vi "GetTestDataHeader.vi"(7 "Boolean":bool, 11 "TESTPLAN ARRAY":string[][](array[string])=[["CUSTOMER P/N:", "SCR-Relay IDM20A", "", "", "", "", "", "", "", "", "", "", "", ""], ["SVI P/N:", "SAB213-143LF", "", "", "", "", "", "", "", "", "", "", "", ""], ["CREATED DATE:", "12-ÁÕ.¤.-14", "", "", "", "", "", "", "", "", "", "", "", ""], ["SW REV.:", "1.000", "", "", "", "", "", "", "", "", "", "", "", ""], ["TEST SEQ REV.:", "1.000", "", "", "", "", "", "", "", "", "", "", "", ""], ["Index", " Step#", "Descriptions", "FailedCode", "Equipment", "Command", "Action ", "Low Limit", "High Limit", "Unit", "Test Loop", "Compensate", "Remarks", "RLY Status"], ["1", "0", "Initial", "", "", "", "STEP", "", "", "", "", "", "", ""], ["2", "", "Clear all relays", "", "RELAY", "@b000t", "TEST", "", "", "", "", "", "", ""], ["3", "1", "Test of Transformer", "", "", "", "STEP", "", "", "", "", "", "", ""], ["4", "", "\"ON RLY1,2 to connect 230VAC to X11-1(L) and X11-3(N)\"", "", "RELAY", "@b001t", "TEST", "", "", "", "", "", "", "\"1,2\""], ["5", "", "Check for 24-30 VAC between X14.1-2.", "", "", "", "STEP", "", "", "", "", "", "", ""], ["6", "", "CONF 34450A to meas. VAC", "", "34450A", "CONF:VOLT:AC 750", "TEST", "", "", "", "", "", "", ""], ["7", "", "\"ON RLY14, 15 to connect 34450A to meas 24VAC\"", "", "RELAY", "@b011t", "TEST", "", "", "", "", "", "", "\"1,2,14,15\""], ["8", "", "Meas 24VAC at X14-1 and X14-2", "1.1", "34450A", "READ?", "TEST", "24", "30", "VAC", "", "", "", ""], ["9", "", "Delay 250mS", "", "DELAY", "250", "TEST", "", "", "", "", "", "", ""], ["10", "2", "Check of PTC-resistors", "", "", "", "STEP", "", "", "", "", "", "", ""], ["11", "", "\"35R at X14-1 & 2, 24VAC at X14-1&2 < 17VAC after 10 sec\"", "2.1", "34450A", "PTC-V35R", "TEST", "10", "15", "Sec", "", "", "35R is connected here in a routine", "\"1,2,14,15,12,13\""], ["12", "", "\"OFF RLY12, 13 to disconnect 35R from X14-1 and X14-2\"", "", "RELAY", "@b010f", "TEST", "", "", "", "", "", "", "\"1,2,14,15\""], ["13", "", "\"OFF RLY14, 15 to disconnect 34450A from X14-1 and X14-2\"", "", "RELAY", "@b011f", "TEST", "", "", "", "", "", "", "\"1,2\""], ["14", "", "CONF 34450A to meas. IAC", "", "34450A", "CONF:CURR:AC 1", "TEST", "", "", "", "", "", "", ""], ["15", "", "\"15R & AC-AMP at X14-1 & 2, I thru 15R <100mA in 15 Sec\"", "2.2", "34450A", "PTC-I15R", "TEST", "15", "20", "Sec", "", "", "15R is connected here in a routine", "\"1,2,16,17,18\""], ["16", "", "\"OFF RLY16,17,18 to disconnect 15R and AC-AMP from X14-1 & 2\"", "", "RELAY", "@b012f", "TEST", "", "", "", "", "", "", "\"1,2\""], ["17", "3", "Test of +34 Volt", "", "", "", "STEP", "", "", "", "", "", "", ""], ["18", "", "CONF 34450A to meas. VDC", "", "34450A", "CONF:VOLT:DC 100", "TEST", "", "", "", "", "", "", ""], ["19", "", "\"ON RLY19,20 to connect 34450A to +34V and GND (X13-8)\"", "", "RELAY", "@b013t", "TEST", "", "", "", "", "", "", "\"1,2,19,20\""], ["20", "", "Meas +34 Volt", "3.1", "34450A", "READ?", "TEST", "30", "38", "VDC", "", "", "", ""], ["21", "", "\"OFF RLY19,20 to disconnect 34450A from +34V and GND (X13-8)\"", "", "RELAY", "@b013t", "TEST", "", "", "", "", "", "", "\"1,2\""], ["22", "", "Test of relays: ", "", "", "", "STEP", "", "", "", "", "", "", ""], ["23", "4", "Test of K1", "", "", "", "STEP", "", "", "", "", "", "", ""], ["24", "", "LED9 is OFF?", "4.1", "MESSAGE", "", "TEST", "1", "1", "", "", "", "", ""], ["25", "", "ON RLY21 to connect 16mA curr to X13-3", "", "RELAY", "@b014t", "TEST", "", "", "", "", "", "", "\"1,2,21\""], ["26", "", "\"ON RLY24,25 to connect 34450A to GND of 16mA CON CKT and X13-1\"", "", "RELAY", "@b017t", "TEST", "", "", "", "", "", "", "\"1,2,21,24,25\""], ["27", "", "Meas VX13-1", "4.2", "34450A", "READ?", "TEST", "-0.5", "0.5", "VDC", "", "", "", ""], ["28", "", "\"OFF RLY24,25 to disconnect 34450A from GND of 16mA CON CKT and X13-1\"", "", "RELAY", "@b017f", "TEST", "", "", "", "", "", "", "\"1,2,21\""], ["29", "", "\"ON RLY24,26 to connect 34450A to GND of 16mA CON CKT and X13-2\"", "", "RELAY", "@b018t", "TEST", "", "", "", "", "", "", "\"1,2,21,24,26\""], ["30", "", "Meas VX13-2", "4.3", "34450A", "READ?", "TEST", "7", "8", "VDC", "", "", "", ""], ["31", "", "\"OFF RLY24,26 to disconnect 34450A from GND of 16mA CON CKT and X13-2\"", "", "RELAY", "@b018f", "TEST", "", "", "", "", "", "", "\"1,2,21\""], ["32", "", "ON RLY5 to activate K1", "", "RELAY", "@b003t", "TEST", "", "", "", "", "", "", "\"1,2,5,21\""], ["33", "", "LED9 is ON?", "4.4", "MESSAGE", "", "TEST", "1", "1", "", "", "", "", ""], ["34", "", "\"ON RLY24,25 to connect 34450A to GND of 16mA CON CKT and X13-1\"", "", "RELAY", "@b017t", "TEST", "", "", "", "", "", "", "\"1,2,5,21,24,25\""], ["35", "", "Meas VX13-1", "4.5", "34450A", "READ?", "TEST", "7", "8", "VDC", "", "", "", ""], ["36", "", "\"OFF RLY24,25 to disconnect 34450A from GND of 16mA CON CKT and X13-1\"", "", "RELAY", "@b017f", "TEST", "", "", "", "", "", "", "\"1,2,5,21\""], ["37", "", "\"ON RLY24,26 to connect 34450A to GND of 16mA CON CKT and X13-2\"", "", "RELAY", "@b018t", "TEST", "", "", "", "", "", "", "\"1,2,5,21,24,26\""], ["38", "", "Meas VX13-2", "4.6", "34450A", "READ?", "TEST", "-0.5", "0.5", "VDC", "", "", "", ""], ["39", "", "\"OFF RLY24,26 to disconnect 34450A from GND of 16mA CON CKT and X13-2\"", "", "RELAY", "@b018f", "TEST", "", "", "", "", "", "", "\"1,2,5,21\""], ["40", "", "OFF RLY21 to disconnect 16mA curr from X13-3", "", "RELAY", "@b014f", "TEST", "", "", "", "", "", "", "\"1,2,5\""], ["41", "", "OFF RLY5 to de-activate K1", "", "RELAY", "@b003f", "TEST", "", "", "", "", "", "", "\"1,2\""], ["42", "5", "Test of K2", "", "", "", "STEP", "", "", "", "", "", "", ""], ["43", "", "LED10 is OFF?", "5.1", "MESSAGE", "", "TEST", "1", "1", "", "", "", "", ""], ["44", "", "ON RLY22 to connect 16mA curr to X13-6", "", "RELAY", "@b015t", "TEST", "", "", "", "", "", "", "\"1,2,22\""], ["45", "", "\"ON RLY24,27 to connect 34450A to GND of 16mA CON CKT and X13-4\"", "", "RELAY", "@b019t", "TEST", "", "", "", "", "", "", "\"1,2,22,24,27\""], ["46", "", "Meas VX13-4", "5.2", "34450A", "READ?", "TEST", "-0.5", "0.5", "VDC", "", "", "", ""], ["47", "", "\"OFF RLY24,27 to disconnect 34450A from GND of 16mA CON CKT and X13-4\"", "", "RELAY", "@b019f", "TEST", "", "", "", "", "", "", "\"1,2,22\""], ["48", "", "\"ON RLY24,28 to connect 34450A to GND of 16mA CON CKT and X13-5\"", "", "RELAY", "@b020t", "TEST", "", "", "", "", "", "", "\"1,2,22,24,28\""], ["49", "", "Meas VX13-5", "5.3", "34450A", "READ?", "TEST", "7", "8", "VDC", "", "", "", ""], ["50", "", "\"OFF RLY24,28 to disconnect 34450A from GND of 16mA CON CKT and X13-5\"", "", "RELAY", "@b020f", "TEST", "", "", "", "", "", "", "\"1,2,22\""], ["51", "", "ON RLY6 to activate K2", "", "RELAY", "@b004t", "TEST", "", "", "", "", "", "", "\"1,2,4,22\""], ["52", "", "LED10 is ON?", "5.4", "MESSAGE", "", "TEST", "1", "1", "", "", "", "", ""], ["53", "", "\"ON RLY24,27 to connect 34450A to GND of 16mA CON CKT and X13-4\"", "", "RELAY", "@b019t", "TEST", "", "", "", "", "", "", "\"1,2,4,22,24,27\""], ["54", "", "Meas VX13-4", "5.2", "34450A", "READ?", "TEST", "7", "8", "VDC", "", "", "", ""], ["55", "", "\"OFF RLY24,27 to disconnect 34450A from GND of 16mA CON CKT and X13-4\"", "", "RELAY", "@b019f", "TEST", "", "", "", "", "", "", "\"1,2,4,22\""], ["56", "", "\"ON RLY24,28 to connect 34450A to GND of 16mA CON CKT and X13-5\"", "", "RELAY", "@b020t", "TEST", "", "", "", "", "", "", "\"1,2,4,22,24,28\""], ["57", "", "Meas VX13-5", "5.3", "34450A", "READ?", "TEST", "-0.5", "0.5", "VDC", "", "", "", ""], ["58", "", "\"OFF RLY24,28 to disconnect 34450A from GND of 16mA CON CKT and X13-5\"", "", "RELAY", "@b020f", "TEST", "", "", "", "", "", "", "\"1,2,4,22\""], ["59", "", "OFF RLY22 to disconnect 16mA curr from X13-6", "", "RELAY", "@b015f", "TEST", "", "", "", "", "", "", "\"1,2,4\""], ["60", "", "OFF RLY6 to de-activate K2", "", "RELAY", "@b004f", "TEST", "", "", "", "", "", "", "\"1,2\""], ["61", "6", "Test of K3", "", "", "", "STEP", "", "", "", "", "", "", ""], ["62", "", "LED11 is OFF?", "6.1", "MESSAGE", "", "TEST", "1", "1", "", "", "", "", ""], ["63", "", "ON RLY23 to connect 16mA curr to X13-8", "", "RELAY", "@b016t", "TEST", "", "", "", "", "", "", "\"1,2,23\""], ["64", "", "\"ON RLY24,29 to connect 34450A to GND of 16mA CON CKT and X13-7\"", "", "RELAY", "@b021t", "TEST", "", "", "", "", "", "", "\"1,2,23,24,29\""], ["65", "", "Meas VX13-7", "6.2", "34450A", "READ?", "TEST", "-0.5", "0.5", "VDC", "", "", "", ""], ["66", "", "\"OFF RLY24,29 to disconnect 34450A from GND of 16mA CON CKT and X13-7\"", "", "RELAY", "@b021f", "TEST", "", "", "", "", "", "", "\"1,2,23\""], ["67", "", "\"ON RLY24,35 to connect 34450A to GND of 16mA CON CKT and X13-9\"", "", "RELAY", "@b029t", "TEST", "", "", "", "", "", "", "\"1,2,23,24,35\""], ["68", "", "Meas VX13-9", "6.3", "34450A", "READ?", "TEST", "7", "8", "VDC", "", "", "", ""], ["69", "", "\"OFF RLY24,35 to disconnect 34450A from GND of 16mA CON CKT and X13-9\"", "", "RELAY", "@b029f", "TEST", "", "", "", "", "", "", "\"1,2,23\""], ["70", "", "ON RLY7 to activate K3", "", "RELAY", "@b005t", "TEST", "", "", "", "", "", "", "\"1,2,3,23\""], ["71", "", "LED11 is ON?", "6.4", "MESSAGE", "", "TEST", "1", "1", "", "", "", "", ""], ["72", "", "\"ON RLY24,29 to connect 34450A to GND of 16mA CON CKT and X13-7\"", "", "RELAY", "@b021t", "TEST", "", "", "", "", "", "", "\"1,2,23,24,29\""], ["73", "", "Meas VX13-7", "6.2", "34450A", "READ?", "TEST", "7", "8", "VDC", "", "", "", ""], ["74", "", "\"OFF RLY24,29 to disconnect 34450A from GND of 16mA CON CKT and X13-7\"", "", "RELAY", "@b021f", "TEST", "", "", "", "", "", "", "\"1,2,23\""], ["75", "", "\"ON RLY24,35 to connect 34450A to GND of 16mA CON CKT and X13-9\"", "", "RELAY", "@b029t", "TEST", "", "", "", "", "", "", "\"1,2,23,24,35\""], ["76", "", "Meas VX13-9", "6.3", "34450A", "READ?", "TEST", "-0.5", "0.5", "VDC", "", "", "", ""], ["77", "", "\"OFF RLY24,35 to disconnect 34450A from GND of 16mA CON CKT and X13-9\"", "", "RELAY", "@b029f", "TEST", "", "", "", "", "", "", "\"1,2,23\""], ["78", "", "OFF RLY23 to disconnect 16mA curr from X13-3", "", "RELAY", "@b016f", "TEST", "", "", "", "", "", "", "\"1,2,3\""], ["79", "", "OFF RLY5 to de-activate K1", "", "RELAY", "@b005f", "TEST", "", "", "", "", "", "", "\"1,2\""], ["80", "", "Test of SC-relay", "", "", "", "STEP", "", "", "", "", "", "", ""], ["81", "7", "Test of TI4", "", "", "", "STEP", "", "", "", "", "", "", ""], ["82", "", "CONF 34450A to meas. VAC", "", "34450A", "CONF:VOLT:AC 750", "TEST", "", "", "", "", "", "", ""], ["83", "", "LED8 is OFF?", "7.1", "MESSAGE", "", "TEST", "1", "1", "", "", "", "", ""], ["84", "", "\"ON RLY30,34 to connect 34450A to X12-1 (L) & X11-3 (N)\"", "", "RELAY", "@b022t", "TEST", "", "", "", "", "", "", "\"1,2,30,34\""], ["85", "", "Meas VX12-1 (L) & X11-3 (N)-NoActivated", "7.2", "34450A", "READ?", "TEST", "0", "10", "VAC", "", "", "", ""], ["86", "", "ON RLY8 to activate TI4 (X15-4 to X15-8)", "", "RELAY", "@b006t", "TEST", "", "", "", "", "", "", "\"1,2,30,34,8\""], ["87", "", "Delay 250mS", "", "DELAY", "250", "TEST", "", "", "", "", "", "", ""], ["88", "", "LED8 is ON?", "7.3", "MESSAGE", "", "TEST", "1", "1", "", "", "", "", ""], ["89", "", "Meas VX12-1 (L) & X11-3 (N)-Activated", "7.4", "34450A", "READ?", "TEST", "210", "250", "VAC", "", "", "", ""], ["90", "", "OFF RLY8 to de-activate TI4 (X15-4 to X15-8)", "", "RELAY", "@b006f", "TEST", "", "", "", "", "", "", "\"1,2,30,34\""], ["91", "", "\"OFF RLY30,34 to disconnect 34450A from X12-1 (L) & X11-3 (N)\"", "", "RELAY", "@b022f", "TEST", "", "", "", "", "", "", "\"1,2\""], ["92", "", "Delay 250mS", "", "DELAY", "250", "TEST", "", "", "", "", "", "", ""], ["93", "8", "Test of TI1", "", "", "", "STEP", "", "", "", "", "", "", ""], ["94", "", "LED5 is OFF?", "8.1", "MESSAGE", "", "TEST", "1", "1", "", "", "", "", ""], ["95", "", "\"ON RLY31,34 to connect 34450A to X12-2 (L) & X11-3 (N)\"", "", "RELAY", "@b023t", "TEST", "", "", "", "", "", "", "\"1,2,31,34\""], ["96", "", "Meas VX12-2 (L) & X11-3 (N)-NoActivated", "8.2", "34450A", "READ?", "TEST", "0", "10", "VAC", "", "", "", ""], ["97", "", "ON RLY9 to activate TI1 (X15-5 to X15-8)", "", "RELAY", "@b007t", "TEST", "", "", "", "", "", "", "\"1,2,31,34,9\""], ["98", "", "Delay 250mS", "", "DELAY", "250", "TEST", "", "", "", "", "", "", ""], ["99", "", "LED5 is ON?", "8.3", "MESSAGE", "", "TEST", "1", "1", "", "", "", "", ""], ["100", "", "Meas VX12-2 (L) & X11-3 (N)-Activated", "8.4", "34450A", "READ?", "TEST", "210", "250", "VAC", "", "", "", ""], ["101", "", "OFF RLY9 to de-activate TI1 (X15-5 to X15-8)", "", "RELAY", "@b007f", "TEST", "", "", "", "", "", "", "\"1,2,31,34\""], ["102", "", "\"OFF RLY30,34 to disconnect 34450A from X12-1 (L) & X11-3 (N)\"", "", "RELAY", "@b023f", "TEST", "", "", "", "", "", "", "\"1,2\""], ["103", "", "Delay 250mS", "", "DELAY", "250", "TEST", "", "", "", "", "", "", ""], ["104", "9", "Test of TI2", "", "", "", "STEP", "", "", "", "", "", "", ""], ["105", "", "LED6 is OFF?", "9.1", "MESSAGE", "", "TEST", "1", "1", "", "", "", "", ""], ["106", "", "\"ON RLY32,34 to connect 34450A to X12-3 (L) & X11-3 (N)\"", "", "RELAY", "@b024t", "TEST", "", "", "", "", "", "", "\"1,2,32,34\""], ["107", "", "Meas VX12-3 (L) & X11-3 (N)-NoActivated", "9.2", "34450A", "READ?", "TEST", "0", "10", "VAC", "", "", "", ""], ["108", "", "ON RLY10 to activate TI2 (X15-6 to X15-8)", "", "RELAY", "@b008t", "TEST", "", "", "", "", "", "", "\"1,2,32,34,10\""], ["109", "", "Delay 250mS", "", "DELAY", "250", "TEST", "", "", "", "", "", "", ""], ["110", "", "LED6 is ON?", "9.3", "MESSAGE", "", "TEST", "1", "1", "", "", "", "", ""], ["111", "", "Meas VX12-3 (L) & X11-3 (N)-Activated", "9.4", "34450A", "READ?", "TEST", "210", "250", "VAC", "", "", "", ""], ["112", "", "OFF RLY10 to de-activate TI2 (X15-6 to X15-8)", "", "RELAY", "@b008f", "TEST", "", "", "", "", "", "", "\"1,2,32,34\""], ["113", "", "\"OFF RLY32,34 to disconnect 34450A from X12-3 (L) & X11-3 (N)\"", "", "RELAY", "@b024f", "TEST", "", "", "", "", "", "", "\"1,2\""], ["114", "", "Delay 250mS", "", "DELAY", "250", "TEST", "", "", "", "", "", "", ""], ["115", "10", "Test of TI3", "", "", "", "STEP", "", "", "", "", "", "", ""], ["116", "", "LED7 is OFF?", "10.1", "MESSAGE", "", "TEST", "1", "1", "", "", "", "", ""], ["117", "", "\"ON RLY33,34 to connect 34450A to X12-4 (L) & X11-3 (N)\"", "", "RELAY", "@b025t", "TEST", "", "", "", "", "", "", "\"1,2,33,34\""], ["118", "", "Meas VX12-4 (L) & X11-3 (N)-NoActivated", "10.2", "34450A", "READ?", "TEST", "0", "10", "VAC", "", "", "", ""], ["119", "", "ON RLY11 to activate TI3 (X15-7 to X15-8)", "", "RELAY", "@b009t", "TEST", "", "", "", "", "", "", "\"1,2,33,34,11\""], ["120", "", "Delay 250mS", "", "DELAY", "250", "TEST", "", "", "", "", "", "", ""], ["121", "", "LED7 is ON?", "10.3", "MESSAGE", "", "TEST", "1", "1", "", "", "", "", ""], ["122", "", "Meas VX12-4 (L) & X11-3 (N)-Activated", "10.4", "34450A", "READ?", "TEST", "210", "250", "VAC", "", "", "", ""], ["123", "", "OFF RLY11 to de-activate TI2 (X15-7 to X15-8)", "", "RELAY", "@b009f", "TEST", "", "", "", "", "", "", "\"1,2,33,34\""], ["124", "", "\"OFF RLY33,34 to disconnect 34450A from X12-4 (L) & X11-3 (N)\"", "", "RELAY", "@b025f", "TEST", "", "", "", "", "", "", "\"1,2\""], ["125", "", "Delay 250mS", "", "DELAY", "250", "TEST", "", "", "", "", "", "", ""], ["126", "", "Clear all relays", "", "RELAY", "@b000t", "TEST", "", "", "", "", "", "", ""], ["127", "", "End of testing", "", "", "", "END", "", "", "", "", "", "", ""]]) -> (3 "TestDataHeader":string)   [LabVIEW 2011]
panel:
  out "element 3":i32
  out "size(s)":i32[](array[numeric])
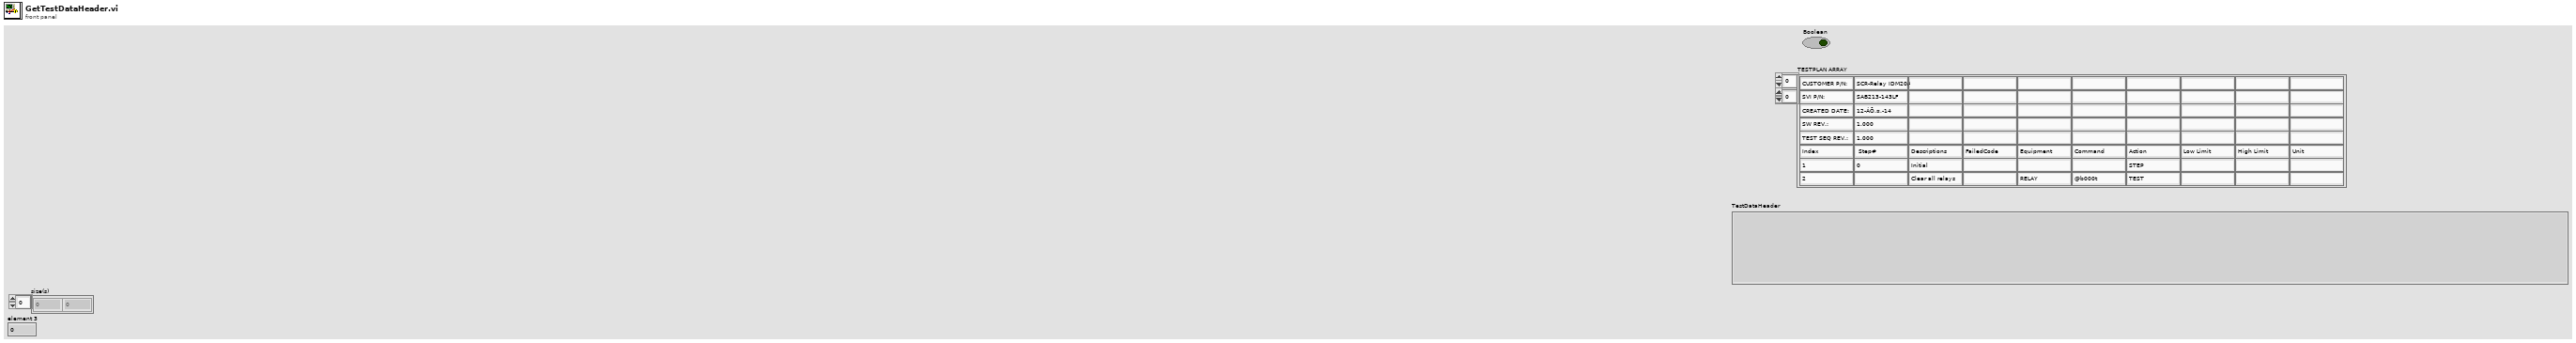
[diagram p1: front panel]
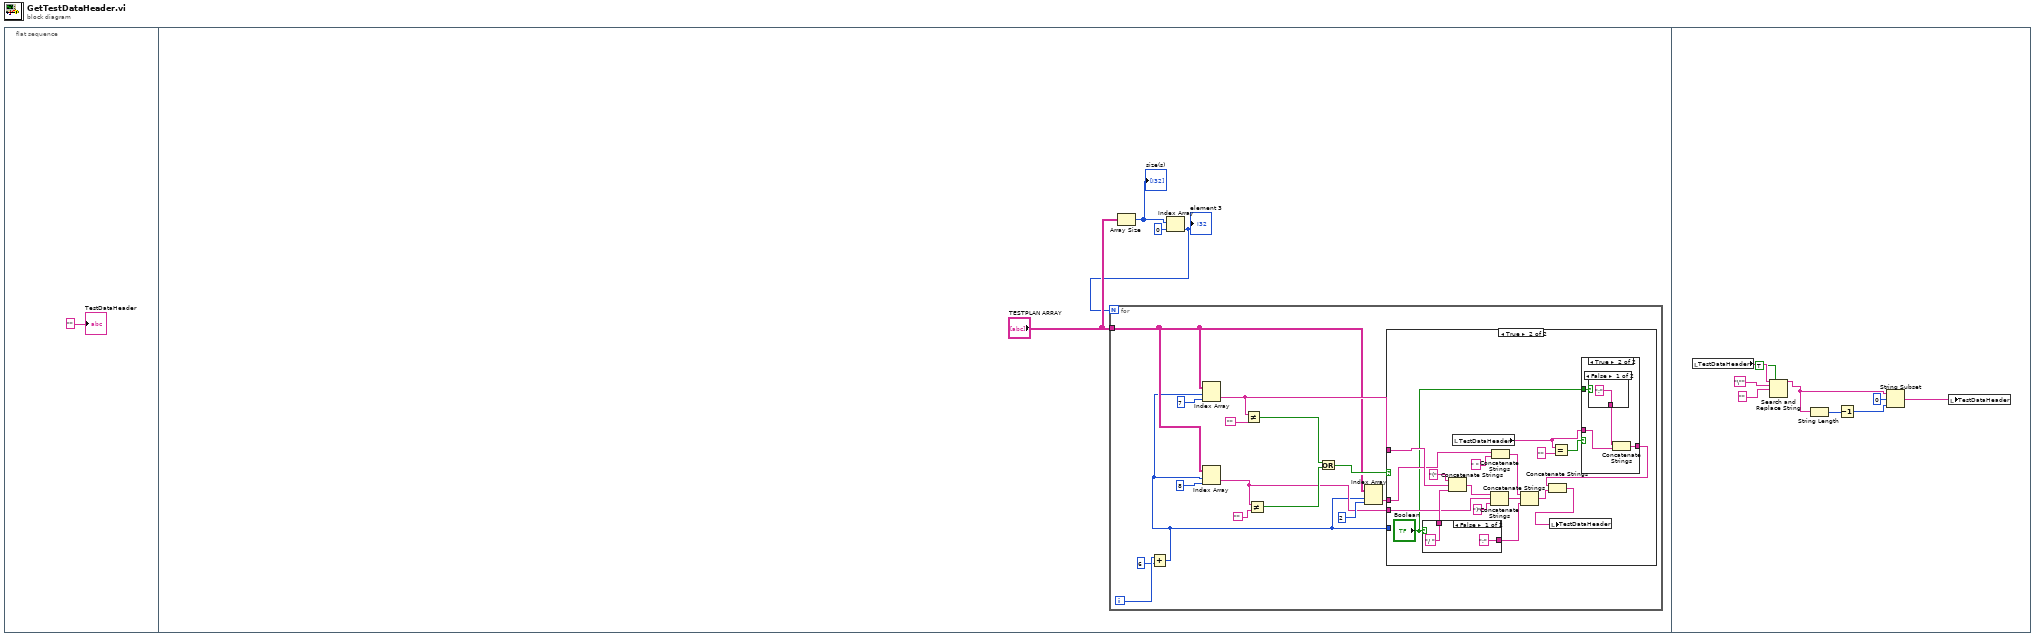
[diagram p0: block diagram]
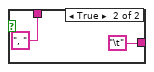
[diagram p3: hidden frame]
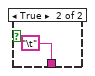
[diagram p5: hidden frame]
diagram:
  n1 = flat-sequence {
    frame #0 {
      "TestDataHeader" <- "" ("String")
    }
    frame #1 {
      n2 = Array Size(array="TESTPLAN ARRAY") -> (size(s)=w4:i32[])
      "size(s)" <- w4
      n3 = Index Array(array=w4, index=0) -> (element=w2:i32)
      "element 3" <- w2
      n4 = for {
        N: w2 -> [_]
        tunnel: "TESTPLAN ARRAY" -> [w9]
        i -> [w8]
        n5 = Add(x=w8, y=6) -> (x+y=w6:i32)
        n6 = Index Array(array=w9, index (row)=w6, index (col)=8 ("disabled index (col)")) -> (element=w10:string)
        n7 = Index Array(array=w9, index (row)=w6, index (col)=7 ("disabled index (col)")) -> (element=w11:string)
        n8 = Not Equal?(x=w11, y="") -> (x != y?=w16:bool)
        n9 = Not Equal?(x=w10, y="") -> (x != y?=w15:bool)
        n10 = Or(x=w16, y=w15) -> (x .or. y?=w14:bool)
        n11 = Index Array(array=w9, index (row)=w6, index (col)=2) -> (element=w12:string)
        n12 = case shown="True" w14 {
          tunnel: w6 -> [_ _]
          tunnel: w12 -> [_ w27]
          tunnel: w11 -> [_ w29]
          tunnel: w10 -> [_ w28]
          frame False {
          }
          frame True {
            n13 = case shown="False" "Boolean" {
              tunnel: ["/ " ", "] -> w31
              tunnel: [";" "\t"] -> w22
              frame False {
              }
              frame True {
              }
            }
            n14 = Concatenate Strings("(", w29, w31) -> (w33:string)
            n15 = local read "TestDataHeader"() -> (w24:string)
            n16 = Concatenate Strings(w33, w28, ")") -> (w36:string)
            n17 = Concatenate Strings(w27, " ") -> (w35:string)
            n18 = Concatenate Strings(w35, w36, w22) -> (w37:string)
            n19 = Equal?(x=w24, y="") -> (x = y?=w26:bool)
            n20 = case shown="True" w26 {
              tunnel: w24 -> [w43 w46]
              tunnel: [w43 w45] -> w23
              tunnel: "Boolean" -> [_ w44]
              frame False {
              }
              frame True {
                n21 = case shown="False" w44 {
                  tunnel: [";" "\t"] -> w47
                  frame False {
                  }
                  frame True {
                  }
                }
                n22 = Concatenate Strings(w47, w46) -> (w45:string)
              }
            }
            n23 = Concatenate Strings(w23, w37) -> (w38:string)
            n24 = local write "TestDataHeader"(w38) -> ()
          }
        }
      }
    }
    frame #2 {
      n25 = local read "TestDataHeader"() -> (w58:string)
      n26 = Search and Replace String(replace all?=TRUE ("replace all? (F)"), input string=w58, search string="\"", replace string="" ("replace string (\"\")")) -> (result string=w51:string)  [unwired: 1 in, 6 out]
      n27 = String Length(string=w51) -> (length=w54:i32)
      n28 = Decrement(x=w54) -> (x-1=w52:i32)
      n29 = String Subset(string=w51, offset (0)=0, length (rest)=w52) -> (substring=w50:string)
      n30 = local write "TestDataHeader"(w50) -> ()
    }
  }
